vi "Has Nested.vi"(8 "error in (no error)":errorcluster, 11 "Module in":refnum<class "Module.lvclass">) -> (0 "error out":errorcluster, 2 "Has Nested":bool, 3 "Module out":refnum<class "Module.lvclass">)   [LabVIEW 2020, in "Volatus.lvlib" / "Module.lvclass"]
uses:
  Module.lvclass
  Module.lvclass/Module.ctl
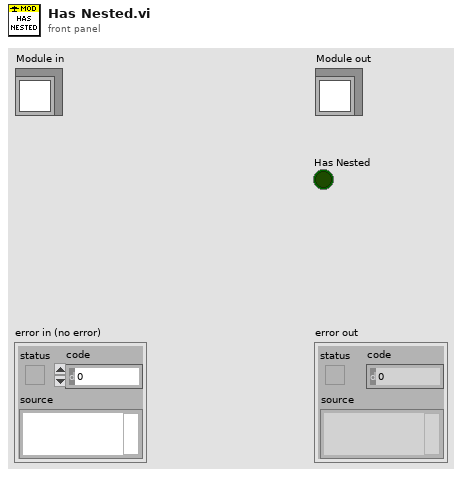
[diagram p1: front panel]
types:
  T1 = typedef "Volatus.lvlib/Module.lvclass/Nested Status.ctl" = cluster{"ID":string, "State":T2}
  T2 = typedef "Volatus.lvlib/Module.lvclass/State.ctl" = enum16{"Unknown", "Launched", "Starting", "Running", "Stopping", "Stopped", "Error - Starting", "Error - Run", "Error - Stopping"}
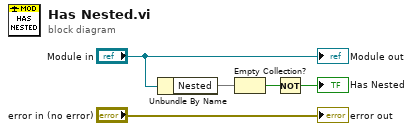
[diagram p0: block diagram]
diagram:
  n1 = Unbundle By Name("Module in") -> ("Nested"=w3:map{refnum<class "MessageQ.lvclass">, T1})
  n2 = Empty Collection?(1:w3) -> (0:w2:bool)
  n3 = Not(x=w2) -> (.not. x?=→"Has Nested":bool)
  "error out" <- "error in (no error)"
  "Module out" <- "Module in"
